vi "Tree Set Default.vi"(8 "error in (no error)":errorcluster, 10 "Node":refnum<data-value>, 11 "Tree DVR in":refnum<data-value>) -> (0 "error out":errorcluster, 3 "Tree DVR out":refnum<data-value>)   [LabVIEW 2010, in "MDSplus.lvlib"]
doc: "Set the default position in the tree."
uses:
  <vilib>/MDSplus/Library/MDSplus.lvlib
  <vilib>/MDSplus/Classes/Tree_Class/Tree.lvclass
  <vilib>/MDSplus/Classes/Data_Class/TreeNode_Class/TreeNode.lvclass
panel:
  out "Node Out":refnum<data-value>
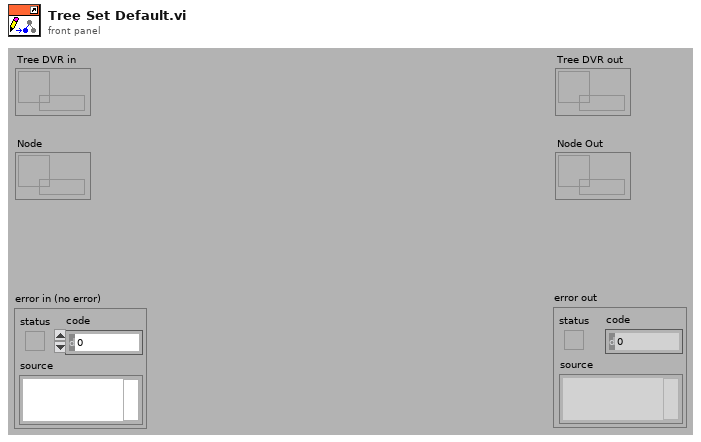
[diagram p1: front panel]
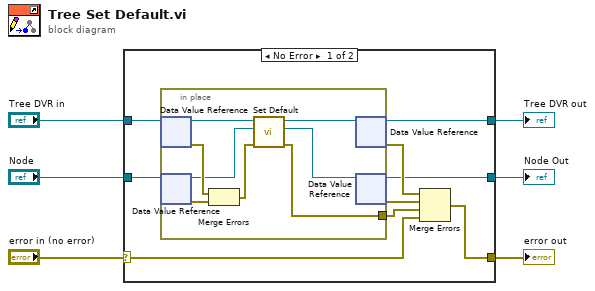
[diagram p0: block diagram]
diagram:
  n1 = case shown="No Error" "error in (no error)" {
    selector: "error in (no error)" -> [w10 w24]
    tunnel: "Tree DVR in" -> [w15 w26]
    tunnel: [w12 w24] -> w6
    tunnel: [w13 w26] -> w3
    tunnel: "Node" -> [w11 w25]
    tunnel: [w7 w25] -> w1
    frame No Error {
      n2 = in-place {
        in-place-border: [w16] -> w8
        n3 = in-place-dvr #1(w15) -> (w23:refnum<class "Tree.lvclass">, w20:errorcluster)
        n4 = in-place-dvr #2(w11) -> (w18:refnum<class "TreeNode.lvclass">, w19:errorcluster)
        n5 = Merge Errors(w20, w19) -> (w21:errorcluster)
        n6 = call-dynamic "Set Default.vi"("error in (no error)"=w21, "Node"=w18, "Tree in"=w23) -> ("error out"=w16:errorcluster, "Node out"=w17:refnum<class "TreeNode.lvclass">, "Tree out"=w22:refnum<class "Tree.lvclass">)  [unwired: 6 in]
        n7 = in-place-dvr #1(w22) -> (w13:refnum<data-value>, w14:errorcluster)
        n8 = in-place-dvr #2(w17) -> (w7:refnum<data-value>, w9:errorcluster)
      }
      n9 = Merge Errors(w14, w9, w8, w10) -> (w12:errorcluster)
    }
    frame Error {
    }
  }
  "error out" <- w6
  "Tree DVR out" <- w3
  "Node Out" <- w1
